vi "Do Search Async.vi"(10 "New Result Event":refnum<user-event>, 11 "Search in":refnum<class "Search.lvclass">) -> ()   [LabVIEW 2020, in "Better Search.lvlib" / "Search.lvclass"]
uses:
  Search.lvclass
  BetterSearch/Search Result.ctl
  Search Result/Search Result.lvclass
  Search.lvclass/Search.ctl
  <vilib>/Utility/traverseref.llb/TRef TravTarget.ctl
  <vilib>/Utility/traverseref.llb/VI Scripting - Traverse.lvlib
  Better Search.lvlib
panel:
  in  "Stop":bool
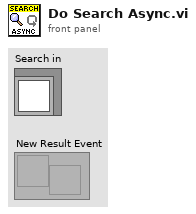
[diagram p1: front panel]
types:
  T1 = enum32{"Invalid", "Standard", "Closed", "Hidden", "Minimized", "Maximized"}
  T2 = typedef "Better Search.lvlib/Search Scope.ctl" = enum16{"Active Target", "Active Project", "Specific Targets", "Active VI", "Active Hierarchy"}
  T3 = typedef "TRef TravTarget.ctl" = enum16{"FP", "BD", "Other"}
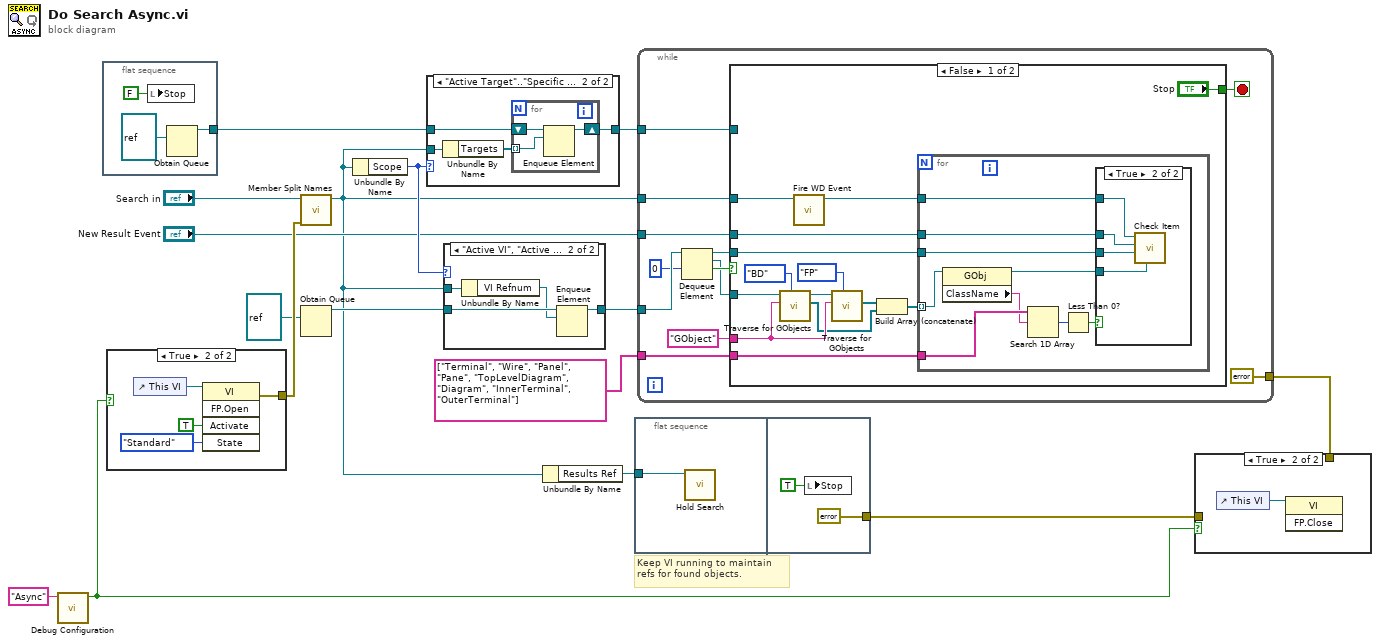
[diagram p0: block diagram]
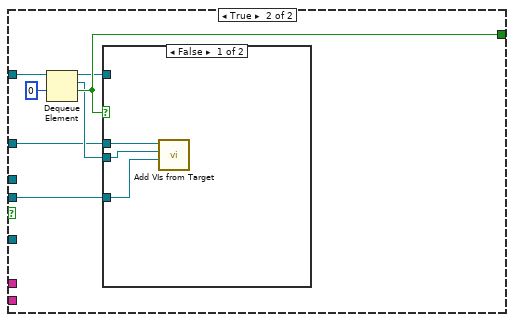
[diagram p5: hidden frame]
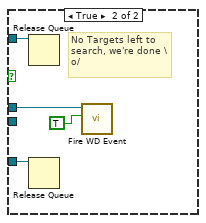
[diagram p6: hidden frame]
diagram:
  # "Keep VI running to maintain refs for found objects."
  n1 = call "Debug Configuration.vi"("Subset (None)"="Async") -> ("Flag?"=w2:bool)  [unwired: 10 in]
  n2 = flat-sequence {
    tunnel: [w18] -> w15
    frame #0 {
      n3 = local write "Stop"(FALSE ("Stop")) -> ()
      n4 = Obtain Queue(element data type=refnum<vi> refnum ("This Application")) -> (queue out=w18:refnum<queue>)  [unwired: 4 in, 2 out]
    }
  }
  n5 = case shown="True" w2 {
    tunnel: [_ w20] -> w16
    frame False {
    }
    frame True {
      n6 = control-ref of="This VI"() -> (w23:refnum<vi>)
      n7 = invoke class="VI" method="FP.Open"(reference=w23, "Activate"=TRUE ("Activate?"), "State"=T1."Standard") -> (error out=w20:errorcluster)  [unwired: 2 in, 4 out]
    }
  }
  n8 = call "Member Split Names.vi"("error in (no error)"=w16, "Search in"="Search in") -> ("Search out"=w5:refnum<class "Search.lvclass">)  [unwired: 8 in, 1 out]
  n9 = Obtain Queue(element data type=refnum<vi> refnum ("type specifier VI Refnum (for type only)")) -> (queue out=w12:refnum<queue>)  [unwired: 4 in, 2 out]
  n10 = Unbundle By Name(w5) -> ("Scope"=w14:T2)
  n11 = case shown="\"Active Target\"..\"Specific Targets\"" w14 {
    tunnel: w15 -> [w24 w27]
    tunnel: w5 -> [_ w26]
    tunnel: [w24 w25] -> w11
    frame Default {
    }
    frame "Active Target".."Specific Targets" {
      n12 = Unbundle By Name(w26) -> ("Targets"=w28:refnum<vi>[])
      n13 = for {
        tunnel: w28 -> [w30] mode=indexing
        shift-right: [w29] -> w25
        shift-left: w27 -> [w31]
        n14 = Enqueue Element(queue=w31, element=w30) -> (queue out=w29:refnum<queue>)  [unwired: 2 in, 2 out]
      }
    }
  }
  n15 = case shown="\"Active VI\", \"Active Hierarchy\"" w14 {
    tunnel: w12 -> [w32 w35]
    tunnel: w5 -> [_ w36]
    tunnel: [w32 w33] -> w10
    frame Default {
    }
    frame "Active VI", "Active Hierarchy" {
      n16 = Unbundle By Name(w36) -> ("VI Refnum"=w34:refnum<vi>)
      n17 = Enqueue Element(queue=w35, element=w34) -> (queue out=w33:refnum<queue>)  [unwired: 2 in, 2 out]
    }
  }
  n18 = Unbundle By Name(w5) -> ("Results Ref"=w7:refnum<data-value>)
  n19 = flat-sequence {
    tunnel: w7 -> [w37]
    tunnel: [errorcluster {"status"=FALSE, "code"=0, "source"=""} ("error constant")] -> w3
    frame #0 {
      n20 = call "Hold Search.vi"("Data Value Reference in"=w37) -> ()  [unwired: 11 in]
    }
    frame #1 {
      n21 = local write "Stop"(TRUE ("Stop")) -> ()
    }
  }
  n22 = while {
    tunnel: w5 -> [w43]
    tunnel: w11 -> [w46]
    tunnel: w10 -> [w51]
    tunnel: string[] ["Terminal", "Wire", "Panel", "Pane", "TopLevelDiagram", "Diagram", "InnerTerminal", "OuterTerminal"] -> [w44]
    tunnel: "New Result Event" -> [w42]
    tunnel: [errorcluster {"status"=FALSE, "code"=0, "source"=""} ("error constant")] -> w4
    stop <- w45 stop-if-true
    n23 = Dequeue Element(queue=w51, timeout in ms (-1)=0) -> (queue out=w47:refnum<queue>, element=w48:refnum<vi>, timed out?=w49:bool)  [unwired: 1 in, 1 out]
    n24 = case shown="False" w49 {
      tunnel: w48 -> [w62 _]
      tunnel: w47 -> [w58 w83]
      tunnel: w46 -> [_ w85]
      tunnel: ["Stop" w82] -> w45
      tunnel: w44 -> [w59 _]
      tunnel: w43 -> [w53 w79]
      tunnel: w42 -> [w57 _]
      tunnel: "GObject" ("Class Name") -> [w56 _]
      frame False {
        n25 = call <vilib>:"Traverse for GObjects.vi"("Traverse Target"=TRef_TravTarget."BD", "Class Name"=w56, "VI Refnum"=w62) -> ("References"=w55:refnum<vi>[], "dup VI Refnum"=w64:refnum<vi>)  [unwired: 5 in, 2 out]
        n26 = call "Fire WD Event.vi"("Search in"=w53) -> ("Search out"=w52:refnum<class "Search.lvclass">)  [unwired: 9 in, 1 out]
        n27 = call <vilib>:"Traverse for GObjects.vi"("Traverse Target"=TRef_TravTarget."FP", "Class Name"=w56, "VI Refnum"=w64) -> ("References"=w61:refnum<vi>[])  [unwired: 5 in, 3 out]
        n28 = Build Array (concatenate)(w61, w55) -> (w60:refnum<vi>[])
        n29 = for {
          tunnel: w60 -> [w74] mode=indexing
          tunnel: w59 -> [w73]
          tunnel: w58 -> [w69]
          tunnel: w52 -> [w68]
          tunnel: w57 -> [w67]
          n30 = property class="GObj"(reference=w74) -> (reference out=w70:refnum<vi>, "ClassName"=w66:string)  [unwired: 1 in, 1 out]
          n31 = Search 1D Array(1D array=w73, element=w66) -> (index of element=w72:i32)  [unwired: 1 in]
          n32 = Less Than 0?(x=w72) -> (x < 0?=w71:bool)
          n33 = case shown="True" w71 {
            tunnel: w70 -> [_ w75]
            tunnel: w69 -> [_ w76]
            tunnel: w68 -> [_ w78]
            tunnel: w67 -> [_ w77]
            frame False {
            }
            frame True {
              n34 = call "Check Item.vi"("GObj Refnum"=w75, "VI Queue"=w76, "New Result Event"=w77, "Search in"=w78) -> ()  [unwired: 6 in, 2 out]
            }
          }
        }
      }
      frame True {
        n35 = Dequeue Element(queue=w85, timeout in ms (-1)=0) -> (queue out=w80:refnum<queue>, element=w81:refnum<vi>, timed out?=w82:bool)  [unwired: 1 in, 1 out]
        n36 = case shown="False" w82 {
          tunnel: w83 -> [w86 w91]
          tunnel: w81 -> [w87 _]
          tunnel: w80 -> [_ w92]
          tunnel: w79 -> [w88 w90]
          frame False {
            n37 = call "Add VIs from Target.vi"("VI Queue"=w86, "Target"=w87, "Search"=w88) -> ()  [unwired: 9 in]
          }
          frame True {
            # "No Targets left to search, we're done \\o/"
            n38 = Release Queue(queue=w92) -> ()  [unwired: 2 in, 3 out]
            n39 = Release Queue(queue=w91) -> ()  [unwired: 2 in, 3 out]
            n40 = call "Fire WD Event.vi"("Completed? (F)"=TRUE ("Completed?"), "Search in"=w90) -> ()  [unwired: 8 in, 2 out]
          }
        }
      }
    }
  }
  n41 = case shown="True" w2 {
    tunnel: w4 -> [_ _]
    tunnel: w3 -> [_ _]
    frame False {
    }
    frame True {
      n42 = control-ref of="This VI"() -> (w93:refnum<vi>)
      n43 = invoke class="VI" method="FP.Close"(reference=w93) -> ()  [unwired: 2 in, 3 out]
    }
  }
